vi "Create HTML Index.vi"() -> ()   [LabVIEW 2011]
panel:
  in  "Folder Path":path=path "D:/inetpub/wwwroot/AguaClaraCode"
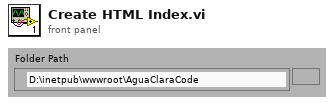
[diagram p1: front panel]
types:
  T1 = enum16{"open", "replace", "create", "open or create", "replace or create", "replace or create with confirmation"}
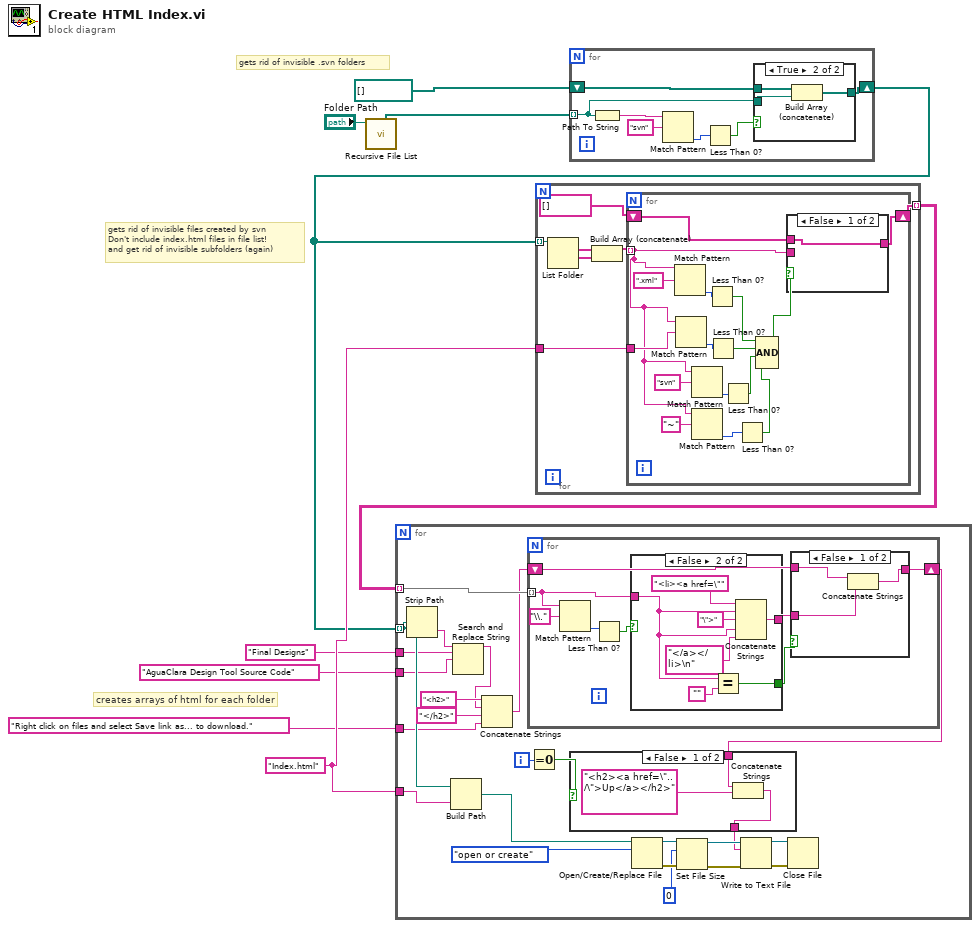
[diagram p0: block diagram]
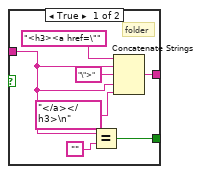
[diagram p3: hidden frame]
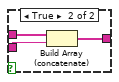
[diagram p6: hidden frame]
diagram:
  w6 = "Index.html" ("name or relative path")
  # "creates arrays of html for each folder"
  # "gets rid of invisible files created by svn\nDon't include index.html files in file list!\nand get rid of invisible subfolders (again)"
  # "gets rid of invisible .svn folders"
  n1 = call <vilib>:"Recursive File List.vi"("Folder Path"="Folder Path") -> ("All Folders"=w7:path[])  [unwired: 6 in, 4 out]
  n2 = for {
    tunnel: w7 -> [w11] mode=indexing
    shift-right: [w13] -> w5
    shift-left: path[] [] -> [w12]
    n3 = Path To String(path=w11) -> (string=w10:string)
    n4 = Match Pattern(string=w10, regular expression="svn") -> (offset past match=w16:i32)  [unwired: 1 in, 3 out]
    n5 = Less Than 0?(x=w16) -> (x < 0?=w14:bool)
    n6 = case shown="True" w14 {
      tunnel: [w17 w20] -> w13
      tunnel: w11 -> [_ w19]
      tunnel: w12 -> [w17 w18]
      frame False {
      }
      frame True {
        n7 = Build Array (concatenate)(w18, w19) -> (w20:path[])
      }
    }
  }
  n8 = for {
    tunnel: w5 -> [w27] mode=indexing
    tunnel: [w24] -> w4 mode=indexing
    tunnel: w6 -> [w23]
    n9 = List Folder(path=w27) -> (filenames=w26:string[], folder names=w21:string[])  [unwired: 3 in, 2 out]
    n10 = Build Array (concatenate)(w26, w21) -> (w22:string[])
    n11 = for {
      tunnel: w22 -> [w28] mode=indexing
      shift-right: [w40] -> w24
      shift-left: string[] [] -> [w41]
      tunnel: w23 -> [w38]
      n12 = Match Pattern(string=w28, regular expression=".xml") -> (offset past match=w42:i32)  [unwired: 1 in, 3 out]
      n13 = Match Pattern(string=w28, regular expression=w38) -> (offset past match=w39:i32)  [unwired: 1 in, 3 out]
      n14 = Match Pattern(string=w28, regular expression="svn") -> (offset past match=w36:i32)  [unwired: 1 in, 3 out]
      n15 = Match Pattern(string=w28, regular expression="~") -> (offset past match=w31:i32)  [unwired: 1 in, 3 out]
      n16 = Less Than 0?(x=w42) -> (x < 0?=w35:bool)
      n17 = Less Than 0?(x=w39) -> (x < 0?=w34:bool)
      n18 = Less Than 0?(x=w36) -> (x < 0?=w33:bool)
      n19 = Less Than 0?(x=w31) -> (x < 0?=w29:bool)
      n20 = Compound Arithmetic op=AND(w35, w34, w33, w29) -> (w32:bool)
      n21 = case shown="False" w32 {
        tunnel: [w44 w47] -> w40
        tunnel: w28 -> [_ w46]
        tunnel: w41 -> [w44 w45]
        frame False {
        }
        frame True {
          n22 = Build Array (concatenate)(w45, w46) -> (w47:string[])
        }
      }
    }
  }
  n23 = for {
    tunnel: w4 -> [w71] mode=indexing
    tunnel: w5 -> [w60] mode=indexing
    tunnel: w6 -> [w70]
    tunnel: "Right click on files and select Save link as... to download." ("string") -> [w56]
    tunnel: "Final Designs" ("string") -> [w53]
    tunnel: "AguaClara Design Tool Source Code" ("string") -> [w52]
    i -> [w51]
    n24 = Strip Path(path=w60) -> (name=w55:string)  [unwired: 1 out]
    n25 = Build Path(base path=w60, name or relative path=w70) -> (appended path=w69:path)
    n26 = Search and Replace String(input string=w55, search string=w53, replace string=w52) -> (result string=w54:string)  [unwired: 5 in, 3 out]
    n27 = Concatenate Strings("<h2>" ("string"), w54, "</h2>" ("string"), w56) -> (w57:string)
    n28 = for {
      tunnel: w71 -> [w79] mode=indexing
      shift-right: [w83] -> w49
      shift-left: w57 -> [w81]
      n29 = Match Pattern(string=w79, regular expression="\\.") -> (offset past match=w78:i32)  [unwired: 1 in, 3 out]
      n30 = Less Than 0?(x=w78) -> (x < 0?=w77:bool)
      n31 = case shown="False" w77 {
        tunnel: [w88 w95] -> w82
        tunnel: w79 -> [w85 w92]
        tunnel: [w84 w91] -> w80
        frame True {
          # "folder"
          n32 = Equal?(x=w85, y="") -> (x = y?=w84:bool)
          n33 = Concatenate Strings("<h3><a href=\"" ("string"), w85, "\">" ("string"), w85, "</a></h3>\n" ("string")) -> (w88:string)
        }
        frame False {
          n34 = Equal?(x=w92, y="") -> (x = y?=w91:bool)
          n35 = Concatenate Strings("<li><a href=\"" ("string"), w92, "\">" ("string"), w92, "</a></li>\n" ("string")) -> (w95:string)
        }
      }
      n36 = case shown="False" w80 {
        tunnel: [w100 w101] -> w83
        tunnel: w82 -> [w99 _]
        tunnel: w81 -> [w98 w101]
        frame False {
          n37 = Concatenate Strings(w98, w99) -> (w100:string)
        }
        frame True {
        }
      }
    }
    n38 = Equal To 0?(x=w51) -> (x = 0?=w50:bool)
    n39 = case shown="False" w50 {
      tunnel: w49 -> [w73 w75]
      tunnel: [w72 w75] -> w48
      frame False {
        n40 = Concatenate Strings(w73, "<h2><a href=\"../\">Up</a></h2>" ("name or relative path")) -> (w72:string)
      }
      frame True {
      }
    }
    n41 = Open/Create/Replace File(file path (use dialog)=w69, operation (0:open)=T1."open or create") -> (refnum out=w65:refnum<file>, error out=w63:errorcluster)  [unwired: 4 in, 1 out]
    n42 = Set File Size(4:w63, 6:i64 0 ("size (in bytes)"), 7:w65) -> (0:w62:errorcluster, 3:w64:refnum<file>)
    n43 = Write to Text File(file (use dialog)=w64, text=w48, error in=w62) -> (refnum out=w66:refnum<file>, error out=w67:errorcluster)  [unwired: 1 in, 1 out]
    n44 = Close File(refnum=w66, error in=w67) -> ()  [unwired: 2 out]
  }
